vi "SailAndRudderArbiter.vi"(6 "JibeSailSuggestion":dbl, 7 "TackingSailSuggestion":dbl, 8 "TurningSailSuggestion":dbl, 9 "LuffToSailSuggestion":dbl, 10 "BalanceRudderSailSugggestion":dbl, 11 "WindToSailLookup":dbl) -> (2 "JibSetpoint":dbl, 3 "MainSailSetpoint":dbl)   [LabVIEW 2012]
panel:
  in  "TurtleModeSailSuggestion":dbl
  in  "TimeOnThisState":i32
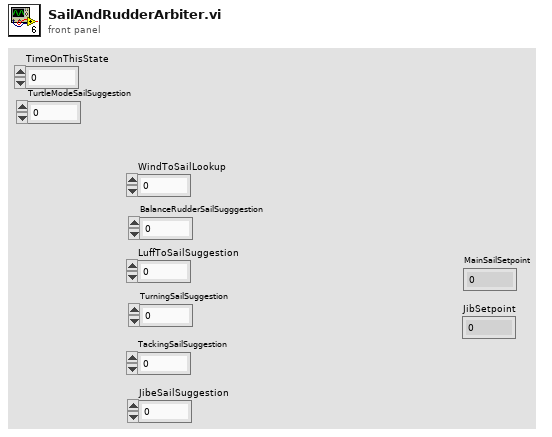
[diagram p1: front panel]
types:
  T1 = enum16{"Straight", "Turning", "Approach Maneuver", "Cross Wind (Tack)", "Cross Wind (Gybe)", "Turtle Mode", ""}
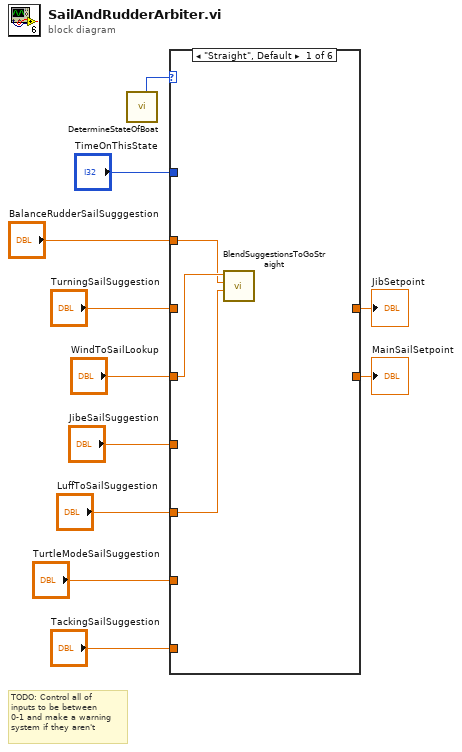
[diagram p0: block diagram]
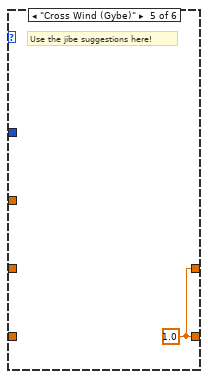
[diagram p5: hidden frame]
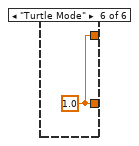
[diagram p6: hidden frame]
diagram:
  # "TODO: Control all of\ninputs to be between\n0-1 and make a warning\nsystem if they aren't"
  n1 = call "DetermineStateOfBoat.vi"() -> ("State of Boat"=w11:T1)  [unwired: 11 in]
  n2 = case shown="\"Straight\", Default" w11 {
    tunnel: [_ w15 w16 _ w17 w18] -> w10
    tunnel: [_ w15 w16 _ w17 w18] -> w9
    tunnel: "JibeSailSuggestion" -> [_ _ _ _ _ _]
    tunnel: "TackingSailSuggestion" -> [_ _ _ _ _ _]
    tunnel: "WindToSailLookup" -> [w14 _ w16 _ _ _]
    tunnel: "TurningSailSuggestion" -> [_ w15 _ _ _ _]
    tunnel: "TimeOnThisState" -> [_ _ _ _ _ _]
    tunnel: "TurtleModeSailSuggestion" -> [_ _ _ _ _ _]
    tunnel: "BalanceRudderSailSugggestion" -> [w13 _ _ _ _ _]
    tunnel: "LuffToSailSuggestion" -> [w12 _ _ _ _ _]
    frame "Straight", Default {
      n3 = call "BlendSuggestionsToGoStraight.vi"("LuffToSailSuggestion"=w12, "BalanceRudderSailSuggestion"=w13, "WindToSailLookup"=w14) -> ()  [unwired: 8 in, 1 out]
    }
    frame "Turning" {
    }
    frame "Approach Maneuver" {
    }
    frame "Cross Wind (Tack)" {
      # "Use the tack suggestions here!"
    }
    frame "Cross Wind (Gybe)" {
      w17 = 1.0 ("MainSailSetpoint")
      # "Use the jibe suggestions here!"
    }
    frame "Turtle Mode" {
      w18 = 1.0 ("MainSailSetpoint")
    }
  }
  "MainSailSetpoint" <- w10
  "JibSetpoint" <- w9
